vi "2-ch2.vi"(3 "this":i32, 4 "button":i32, 5 "shift in":bool, 6 "settings in":T1={"Auto1"=TRUE, "Auto2"=TRUE, "Rel1"=TRUE, "Rel2"=TRUE, "Filt1"=TRUE, "Filt2"=TRUE, "Rate"=enum."Med", "Range1"=enum."10mV", "Range2"=enum."100mV", "Filt3"=TRUE, "Filt4"=TRUE, "Rel temp"=TRUE, "Analog1"=FALSE, "Analog2"=FALSE, "Analog temp"=FALSE, "Digital1"=TRUE, "Digital2"=TRUE, "Digital temp "=TRUE, "Window1"=enum."0,01%", "Window2"=enum."0,01%", "Window temp"=enum."0,01%", "RDGS1"="010", "RDGS2"="010", "RDGS temp"="010", "Type_type1"=TRUE, "Type_type2"=TRUE, "Type_type temp"=TRUE, "LSync"=FALSE, "Unit"=enum."C", "Sens"=TRUE, "Type tcoupl"=enum."J", "Junc"=TRUE}) -> (0 "next state":i32, 1 "shift out":bool, 2 "settings out":T1)   [LabVIEW 2017]
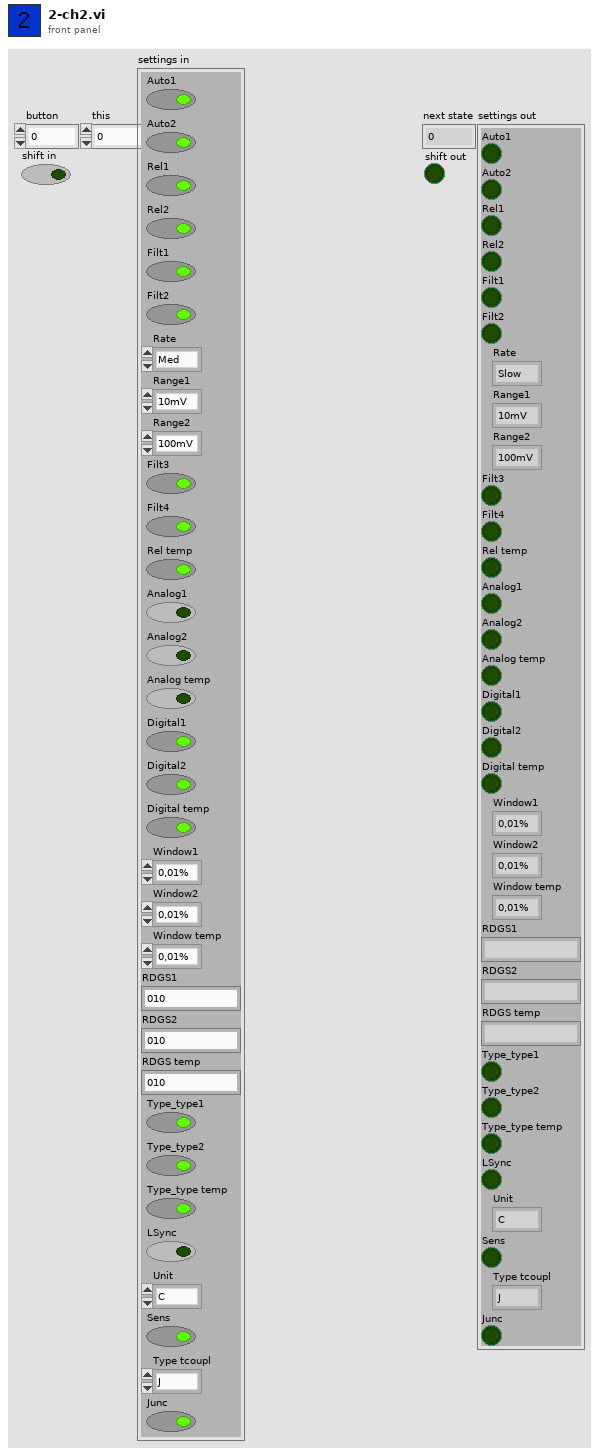
[diagram p1: front panel]
types:
  T1 = cluster{"Auto1":bool, "Auto2":bool, "Rel1":bool, "Rel2":bool, "Filt1":bool, "Filt2":bool, "Rate":enum16{"Slow", "Med", "Fast"}, "Range1":enum16{"10mV", "100mV", "1V", "10V", "100V"}, "Range2":enum16{"100mV", "1V", "10V"}, "Filt3":bool, "Filt4":bool, "Rel temp":bool, "Analog1":bool, "Analog2":bool, "Analog temp":bool, "Digital1":bool, "Digital2":bool, "Digital temp ":bool, "Window1":enum16{"0,01%", "0,1%", "1%", "10%", "None"}, "Window2":enum16{"0,01%", "0,1%", "1%", "10%", "None"}, "Window temp":enum16{"0,01%", "0,1%", "1%", "10%", "None"}, "RDGS1":string, "RDGS2":string, "RDGS temp":string, "Type_type1":bool, "Type_type2":bool, "Type_type temp":bool, "LSync":bool, "Unit":enum16{"C", "K", "F"}, "Sens":bool, "Type tcoupl":enum16{"J", "K", "T", "E", "R", "S", "B", "N"}, "Junc":bool}
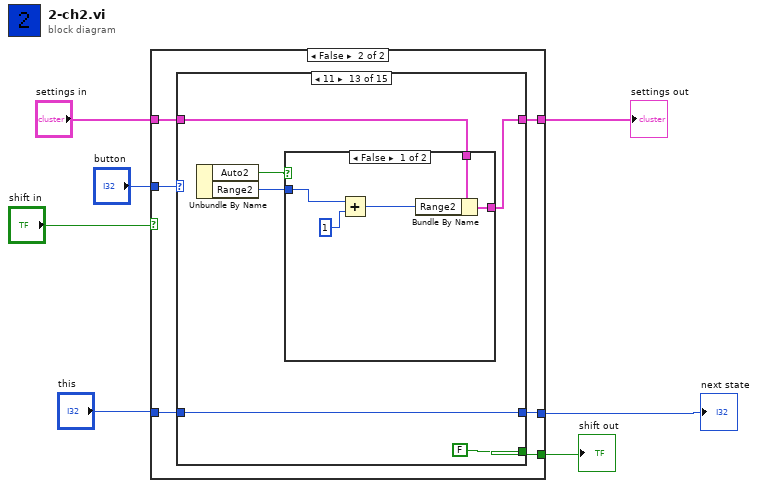
[diagram p0: block diagram]
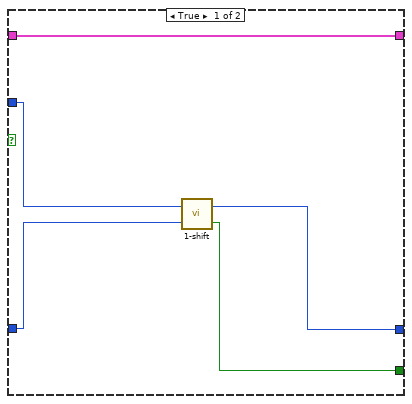
[diagram p2: hidden frame]
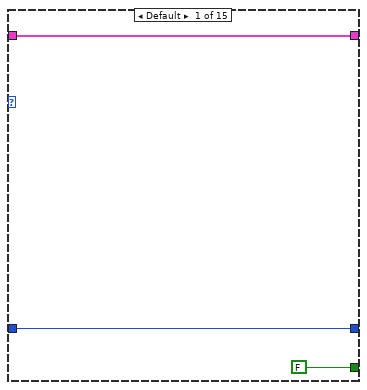
[diagram p3: hidden frame]
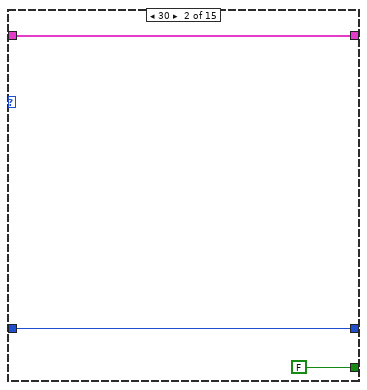
[diagram p4: hidden frame]
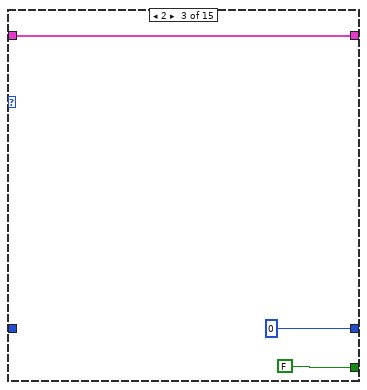
[diagram p5: hidden frame]
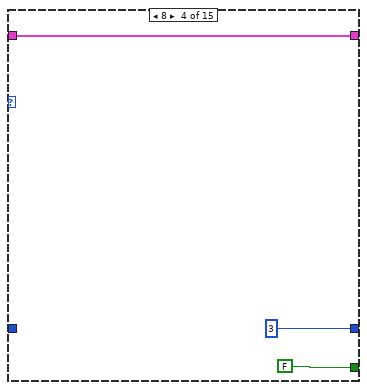
[diagram p6: hidden frame]
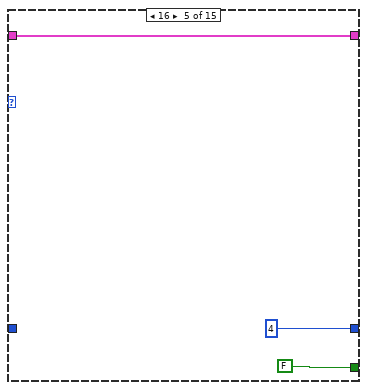
[diagram p7: hidden frame]
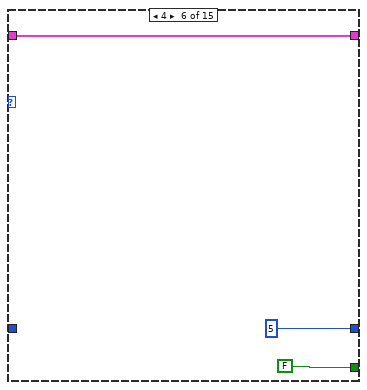
[diagram p8: hidden frame]
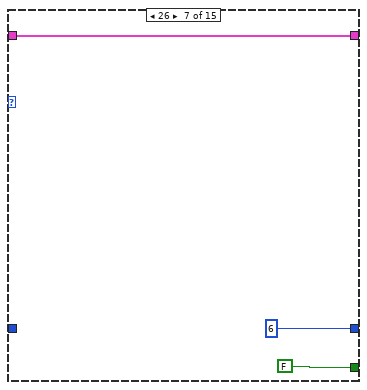
[diagram p9: hidden frame]
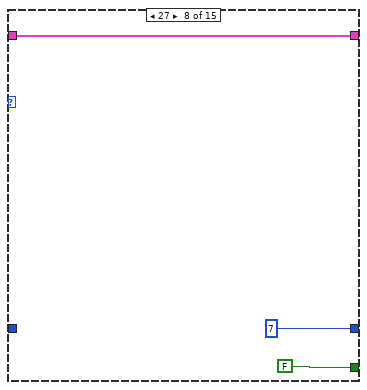
[diagram p10: hidden frame]
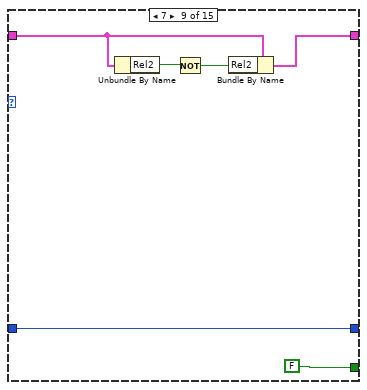
[diagram p11: hidden frame]
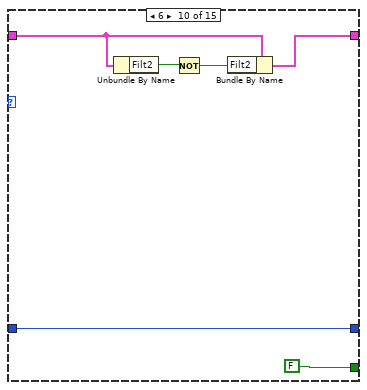
[diagram p12: hidden frame]
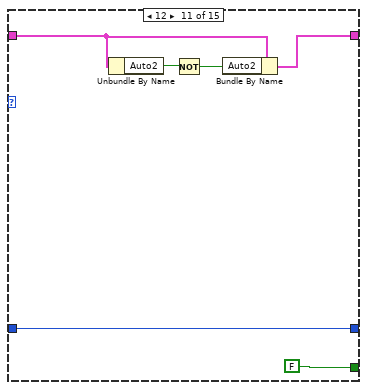
[diagram p13: hidden frame]
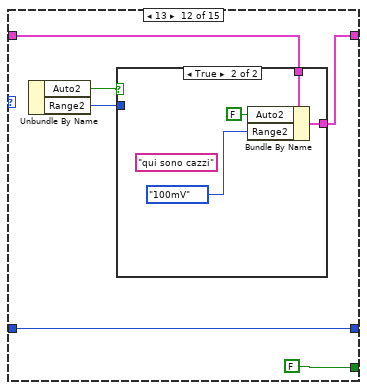
[diagram p14: hidden frame]
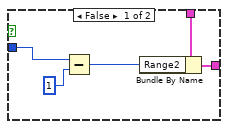
[diagram p15: hidden frame]
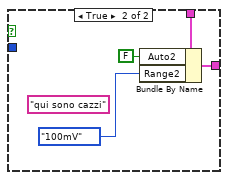
[diagram p16: hidden frame]
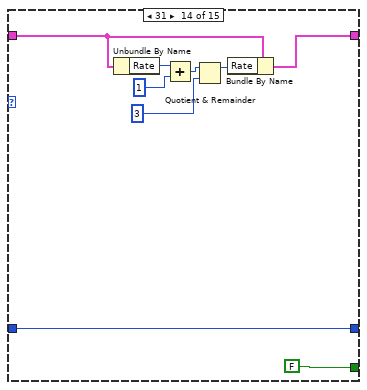
[diagram p17: hidden frame]
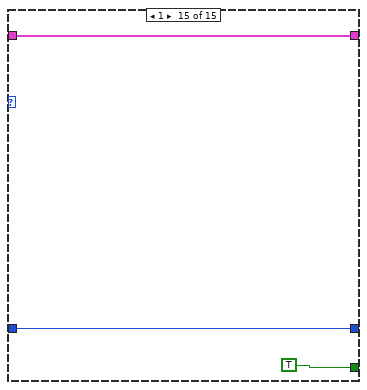
[diagram p18: hidden frame]
diagram:
  n1 = case shown="False" "shift in" {
    tunnel: "button" -> [w12 w18]
    tunnel: [w11 w17] -> w5
    tunnel: "this" -> [w10 w16]
    tunnel: [w8 w15] -> w3
    tunnel: "settings in" -> [w9 w14]
    tunnel: [w9 w13] -> w1
    frame True {
      n2 = call "1-shift.vi"("this"=w10, "button"=w12) -> ("shift"=w8:bool, "next state"=w11:i32)
    }
    frame False {
      n3 = case shown="11" w18 {
        tunnel: [w20 w23 0 3 4 5 6 7 w47 w53 w59 w65 w80 w98 w102] -> w17
        tunnel: w16 -> [w20 w23 _ _ _ _ _ _ w47 w53 w59 w65 w80 w98 w102]
        tunnel: [FALSE ("shift") FALSE ("shift") FALSE ("shift") FALSE ("shift") FALSE ("shift") FALSE ("shift") FALSE ("shift") FALSE ("shift") FALSE ("shift") FALSE ("shift") FALSE ("shift") FALSE ("shift") FALSE ("shift") FALSE ("shift") TRUE ("shift")] -> w15
        tunnel: w14 -> [w21 w24 w25 w28 w31 w34 w37 w40 w44 w50 w56 w62 w77 w97 w100]
        tunnel: [w21 w24 w25 w28 w31 w34 w37 w40 w43 w49 w55 w61 w76 w96 w100] -> w13
        frame Default {
        }
        frame 30 {
        }
        frame 2 {
        }
        frame 8 {
        }
        frame 16 {
        }
        frame 4 {
        }
        frame 26 {
        }
        frame 27 {
        }
        frame 7 {
          n4 = Unbundle By Name(w44) -> ("Rel2"=w46:bool)
          n5 = Not(x=w46) -> (.not. x?=w45:bool)
          n6 = Bundle By Name(cluster=w44, "Rel2"=w45) -> (w43:T1)
        }
        frame 6 {
          n7 = Unbundle By Name(w50) -> ("Filt2"=w52:bool)
          n8 = Not(x=w52) -> (.not. x?=w51:bool)
          n9 = Bundle By Name(cluster=w50, "Filt2"=w51) -> (w49:T1)
        }
        frame 12 {
          n10 = Unbundle By Name(w56) -> ("Auto2"=w58:bool)
          n11 = Not(x=w58) -> (.not. x?=w57:bool)
          n12 = Bundle By Name(cluster=w56, "Auto2"=w57) -> (w55:T1)
        }
        frame 13 {
          n13 = Unbundle By Name() -> ("Auto2"=w63:bool, "Range2"=w64:enum16{"100mV", "1V", "10V"})  [unwired: 1 in]
          n14 = case shown="True" w63 {
            tunnel: [w67 w75] -> w61
            tunnel: w64 -> [w70 _]
            tunnel: w62 -> [w68 w73]
            frame False {
              n15 = Subtract(x=w70, y=1) -> (x-y=w69:i32)
              n16 = Bundle By Name(cluster=w68, "Range2"=w69) -> (w67:T1)
            }
            frame True {
              (unwired) "qui sono cazzi"
              n17 = Bundle By Name(cluster=w73, "Auto2"=FALSE ("Auto1"), "Range2"=enum16{"100mV", "1V", "10V"}."100mV") -> (w75:T1)
            }
          }
        }
        frame 11 {
          n18 = Unbundle By Name() -> ("Auto2"=w78:bool, "Range2"=w79:enum16{"100mV", "1V", "10V"})  [unwired: 1 in]
          n19 = case shown="False" w78 {
            tunnel: [w82 w90] -> w76
            tunnel: w79 -> [w85 _]
            tunnel: w77 -> [w83 w88]
            frame False {
              n20 = Add(x=w85, y=1) -> (x+y=w84:i32)
              n21 = Bundle By Name(cluster=w83, "Range2"=w84) -> (w82:T1)
            }
            frame True {
              (unwired) "qui sono cazzi"
              n22 = Bundle By Name(cluster=w88, "Auto2"=FALSE ("Auto1"), "Range2"=enum16{"100mV", "1V", "10V"}."100mV") -> (w90:T1)
            }
          }
        }
        frame 31 {
          n23 = Unbundle By Name(w97) -> ("Rate"=w95:enum16{"Slow", "Med", "Fast"})
          n24 = Add(x=w95, y=1) -> (x+y=w93:i32)
          n25 = Quotient & Remainder(x=w93, y=3) -> (x-y*floor(x/y)=w92:i32)  [unwired: 1 out]
          n26 = Bundle By Name(cluster=w97, "Rate"=w92) -> (w96:T1)
        }
        frame 1 {
        }
      }
    }
  }
  "next state" <- w5
  "shift out" <- w3
  "settings out" <- w1
